vi "CRYUpdate Jump Info.vi"(8 "SourceCount":i32, 9 "MoveCount":i32, 10 "Step number Selected":i32, 11 "Action":T2(ring)) -> (0 "Jump State Out":T1(array[cluster]), 2 "Canceled?":bool)   [LabVIEW 2013]
uses:
  CRYProject Editor Global.vi
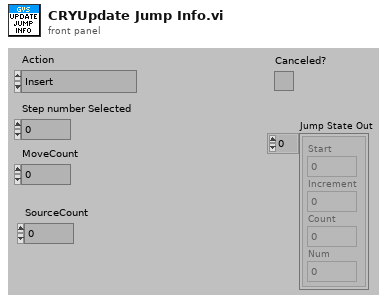
[diagram p1: front panel]
types:
  T1 = cluster{"Start":dbl, "Increment":dbl, "Count":i32, "Num":i32}[]
  T2 = enum16{"Insert", "Remove", "Move up", "Move down"}
  T3 = typedef "CRYTS.ctl" = cluster{"No.TS":u16, "TS File Path":path, "TS Name":string, "EditStepName":string, "Steps":T4[], "New State":bool, "Change State":bool, "Flattened CurveLib Data":string, "Document Data":string, "EditStepNo":u16, "Operator Start File":string, "Sequence Type":string, "Sequence Language":string}
  T4 = typedef "CRYStep.ctl" = cluster{"No.VI":i32, "Category":string, "StepName":string, "Seq setup flattened":string, "Comment":string, "Steps config.":bool[], "Jump config":i32[], "Start":dbl, "Increment":dbl, "Name":string, "Unit":string, "Y data":u16, "Y prefix":string, "Y dB ref":dbl, "Y unit":string, "Repeat State Array":cluster{"Start":dbl, "Increment":dbl, "Count":i32, "Num":i32}[]}
  T5 = enum16{"OK", "Yes", "YesNo", "YesNoCancel", "ReplaceAppend"}
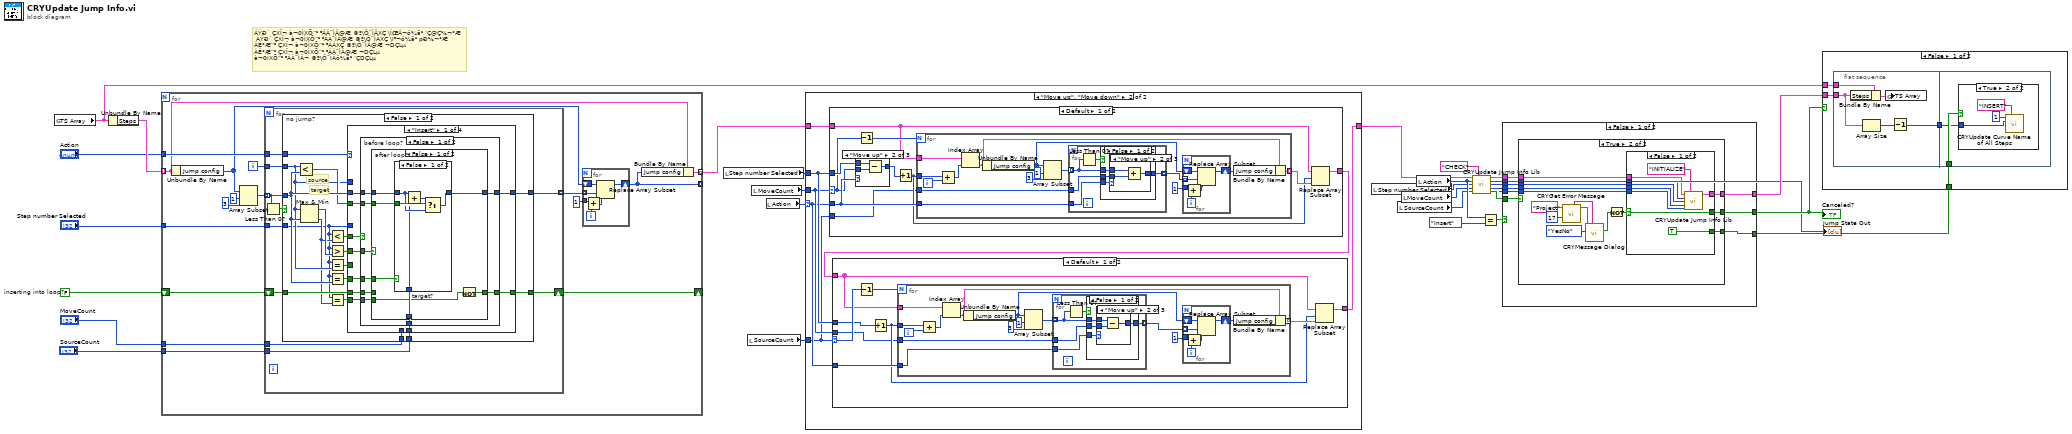
[diagram p0: block diagram]
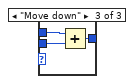
[diagram p4: hidden frame]
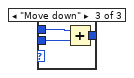
[diagram p8: hidden frame]
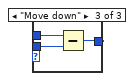
[diagram p10: hidden frame]
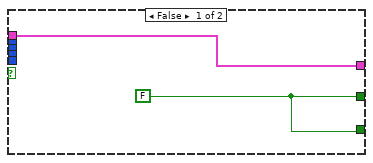
[diagram p15: hidden frame]
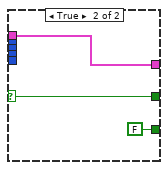
[diagram p16: hidden frame]
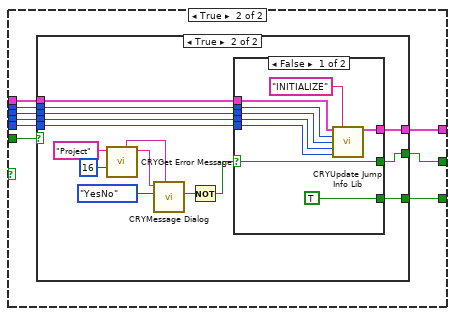
[diagram p17: hidden frame]
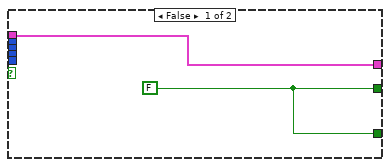
[diagram p18: hidden frame]
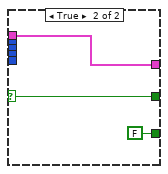
[diagram p19: hidden frame]
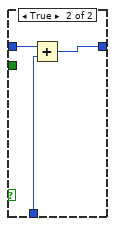
[diagram p20: hidden frame]
diagram:
  w24 = FALSE  # inserting into loop?
  # "ÁÝÐ´ ÇXÎ¬ à¬0ÌXÕ”² ³ÁÀ¨ÌÂ@Æ ©º\\Ô¨ÌÂXÇ \\ÍŒÁ¬ô¼ä² ‘Ç@Ç½¬°Æ\n ÁÝÐ´ ÇXÎ¬ à¬0ÌXÕ”² ³ÁÀ¨ÌÂ@Æ ©º\\Ô¨ÌÂXÇ \\Í³¬ô¼ä² pÐ½¬°Æ\nÀÉ°Æ”² ÇXÎ¬ à¬0ÌXÕ”² ³ÁÀXÇ ©º\\Ô¨ÌÂ@Æ ¬DÇLµ\nÀÉ°Æ”² ÇXÎ¬ à¬0ÌXÕ”² ³ÁÀ¨ÌÂ@Æ ¬DÇLµ\nà¬0ÌXÕ”² ³ÁÀ¨ÌÂ¬ ©º\\Ô¨ÌÂô¼ä² ‘ÇDÇLµ"
  n1 = global read "CRYProject Editor Global.vi" "TS Array"() -> (w23:T3)
  n2 = Unbundle By Name(w23) -> ("Steps"=w17:T4[])
  n3 = for {
    tunnel: "Step number Selected" -> [w39]
    tunnel: "Action" -> [w38]
    tunnel: [w29] -> _ mode=indexing
    tunnel: "SourceCount" -> [w35]
    shift-right: [w33] -> _
    shift-left: w24 -> [w34]
    tunnel: w17 -> [w30] mode=indexing
    tunnel: [w28] -> w21 mode=indexing
    tunnel: "MoveCount" -> [w27]
    i -> [w40]
    n4 = Unbundle By Name(w30) -> ("Jump config"=w31:i32[])
    n5 = Array Subset(array=w31, index=1, length=3) -> (w32:i32[])
    n6 = for {
      tunnel: w32 -> [w57] mode=indexing
      tunnel: w40 -> [w56]
      tunnel: w39 -> [w55]
      tunnel: w38 -> [w54]
      tunnel: [w53] -> w36 mode=indexing
      tunnel: w35 -> [w52]
      shift-right: [w51] -> w33
      shift-left: w34 -> [w50]
      tunnel: w27 -> [w49]
      n7 = Less Than 0?(x=w57) -> (x < 0?=w58:bool)
      n8 = case "no jump?" shown="False" w58 {
        tunnel: w57 -> [w70 w315]
        tunnel: w56 -> [w66 _]
        tunnel: w55 -> [w61 _]
        tunnel: w54 -> [w75 _]
        tunnel: [w73 w315] -> w53
        tunnel: w52 -> [w65 _]
        tunnel: [w64 w314] -> w51
        tunnel: w50 -> [w63 w314]
        tunnel: w49 -> [w59 _]
        frame False {
          # "target"
          # "source"
          n9 = Less?(x=w66, y=w70) -> (x < y?=w67:bool)
          n10 = Max & Min(x=w66, y=w70) -> (max(x,y)=w71:i32, min(x,y)=w62:i32)
          n11 = Less?(x=w61, y=w62) -> (x < y?=w74:bool)
          n12 = Greater?(x=w61, y=w71) -> (0:w72:bool)
          n13 = Equal?(x=w61, y=w66) -> (x = y?=w68:bool)
          n14 = Equal?(x=w61, y=w70) -> (x = y?=w69:bool)
          n15 = Equal?(x=w61, y=w62) -> (x = y?=w60:bool)
          n16 = case shown="\"Insert\"" w75 {
            tunnel: w74 -> [w85 w124 w165 w245]
            tunnel: w70 -> [w84 w123 w164 w244]
            tunnel: [w83 w122 w163 w243] -> w73
            tunnel: w72 -> [w82 w121 w162 w242]
            tunnel: w69 -> [w81 w120 w161 w241]
            tunnel: w68 -> [_ w119 w160 w240]
            tunnel: w67 -> [w80 w118 w159 w239]
            tunnel: w61 -> [_ _ w158 w238]
            tunnel: w66 -> [_ _ w157 w237]
            tunnel: w65 -> [w79 w116 w154 w234]
            tunnel: [w78 w117 w156 w236] -> w64
            tunnel: w63 -> [w77 w117 w156 w236]
            tunnel: w60 -> [w76 _ _ _]
            tunnel: w59 -> [_ _ w155 w235]
            frame "Insert" {
              n17 = case "before loop?" shown="False" w85 {
                tunnel: w84 -> [w93 w115]
                tunnel: [w92 w113] -> w83
                tunnel: w82 -> [w94 _]
                tunnel: w81 -> [w91 _]
                tunnel: w80 -> [w90 _]
                tunnel: w79 -> [w89 w114]
                tunnel: [w88 w112] -> w78
                tunnel: w77 -> [w87 w112]
                tunnel: w76 -> [w86 _]
                frame False {
                  n18 = case "after loop?" shown="False" w94 {
                    tunnel: [w100 w111] -> w92
                    tunnel: w93 -> [w99 w111]
                    tunnel: w91 -> [w101 _]
                    tunnel: w90 -> [w98 _]
                    tunnel: w89 -> [w97 _]
                    tunnel: [w95 w110] -> w88
                    tunnel: w87 -> [_ w110]
                    tunnel: w86 -> [w96 _]
                    frame False {
                      n19 = case "target?" shown="False" w101 {
                        tunnel: [w106 w108] -> w100
                        tunnel: w99 -> [w104 w109]
                        tunnel: w98 -> [w105 _]
                        tunnel: w97 -> [w102 w107]
                        frame False {
                          n20 = Add(x=w104, y=w102) -> (x+y=w103:i32)
                          n21 = Select(t=w103, s=w105, f=w104) -> (s? t:f=w106:i32)
                        }
                        frame True {
                          n22 = Add(x=w109, y=w107) -> (x+y=w108:i32)
                        }
                      }
                      n23 = Not(x=w96) -> (.not. x?=w95:bool)
                    }
                    frame True {
                    }
                  }
                }
                frame True {
                  n24 = Add(x=w115, y=w114) -> (x+y=w113:i32)
                }
              }
            }
            frame "Remove" {
              n25 = case "before loop?" shown="False" w124 {
                tunnel: w123 -> [w130 w153]
                tunnel: [w129 w151] -> w122
                tunnel: w121 -> [w131 _]
                tunnel: w120 -> [w128 _]
                tunnel: w119 -> [w127 _]
                tunnel: w118 -> [w126 _]
                tunnel: w116 -> [w125 w152]
                frame False {
                  n26 = case "after loop?" shown="False" w131 {
                    tunnel: [w136 w150] -> w129
                    tunnel: w130 -> [w135 w150]
                    tunnel: w128 -> [w137 _]
                    tunnel: w127 -> [w134 _]
                    tunnel: w126 -> [w133 _]
                    tunnel: w125 -> [w132 _]
                    frame False {
                      n27 = case "target?" shown="False" w137 {
                        tunnel: [w141 -1] -> w136
                        tunnel: w135 -> [w142 _]
                        tunnel: w134 -> [w140 _]
                        tunnel: w133 -> [w139 _]
                        tunnel: w132 -> [w138 _]
                        frame False {
                          n28 = case "source?" shown="False" w140 {
                            tunnel: [w146 -1] -> w141
                            tunnel: w142 -> [w145 _]
                            tunnel: w139 -> [w147 _]
                            tunnel: w138 -> [w144 _]
                            frame False {
                              n29 = Decrement(x=w145) -> ()  [unwired: 1 out]
                              n30 = Subtract(x=w145, y=w144) -> (x-y=w143:i32)
                              n31 = Select(t=w143, s=w147, f=w145) -> (s? t:f=w146:i32)
                            }
                            frame True {
                            }
                          }
                        }
                        frame True {
                        }
                      }
                    }
                    frame True {
                    }
                  }
                }
                frame True {
                  n32 = Decrement(x=w153) -> ()  [unwired: 1 out]
                  n33 = Subtract(x=w153, y=w152) -> (x-y=w151:i32)
                }
              }
            }
            frame "Move up" {
              n34 = case "before loop?" shown="False" w165 {
                tunnel: w164 -> [w174 w233]
                tunnel: [w173 w233] -> w163
                tunnel: w162 -> [w175 _]
                tunnel: w161 -> [w172 _]
                tunnel: w160 -> [w171 _]
                tunnel: w159 -> [w170 _]
                tunnel: w158 -> [w169 _]
                tunnel: w157 -> [w168 _]
                tunnel: w155 -> [w167 _]
                tunnel: w154 -> [w166 _]
                frame False {
                  n35 = case "after loop?" shown="False" w175 {
                    tunnel: [w183 w227] -> w173
                    tunnel: w174 -> [w182 w226]
                    tunnel: w172 -> [w184 _]
                    tunnel: w171 -> [w181 _]
                    tunnel: w170 -> [w180 _]
                    tunnel: w169 -> [w178 w230]
                    tunnel: w168 -> [w179 _]
                    tunnel: w167 -> [w177 w223]
                    tunnel: w166 -> [w176 w224]
                    frame False {
                      n36 = case "target?" shown="False" w184 {
                        tunnel: [w191 w215] -> w183
                        tunnel: w182 -> [w192 w214]
                        tunnel: w181 -> [w190 _]
                        tunnel: w180 -> [w189 _]
                        tunnel: w179 -> [w188 w219]
                        tunnel: w178 -> [w187 _]
                        tunnel: w177 -> [w186 w211]
                        tunnel: w176 -> [w185 w212]
                        frame False {
                          n37 = case "source?" shown="False" w190 {
                            tunnel: [w199 w204] -> w191
                            tunnel: w192 -> [w197 w205]
                            tunnel: w189 -> [_ _]
                            tunnel: w188 -> [_ w206]
                            tunnel: w187 -> [w198 _]
                            tunnel: w186 -> [w194 _]
                            tunnel: w185 -> [w195 _]
                            frame False {
                              n38 = Decrement(x=w198) -> (x-1=w201:i32)
                              n39 = Increment(x=w197) -> ()  [unwired: 1 out]
                              n40 = Equal?(x=w201, y=w197) -> (x = y?=w200:bool)
                              n41 = case shown="Default" w195 {
                                selector: w195 -> [w202 _]
                                tunnel: [w202 w203] -> w193
                                tunnel: w194 -> [_ w203]
                                frame Default {
                                }
                                frame 1 {
                                }
                              }
                              n42 = Add(x=w197, y=w193) -> (x+y=w196:i32)
                              n43 = Select(t=w196, s=w200, f=w197) -> (s? t:f=w199:i32)
                            }
                            frame True {
                              n44 = Decrement(x=w206) -> (x-1=w209:i32)
                              n45 = Equal?(x=w209, y=w205) -> (x = y?=w207:bool)
                              n46 = Select(t=-1, s=w207, f=w205) -> (s? t:f=w204:i32)
                            }
                          }
                        }
                        frame True {
                          n47 = Increment(x=w219) -> (x+1=w218:i32)
                          n48 = Equal?(x=w218, y=w214) -> (x = y?=w216:bool)
                          n49 = Decrement(x=w214) -> ()  [unwired: 1 out]
                          n50 = case shown="1" w212 {
                            selector: w212 -> [w220 _]
                            tunnel: [w220 w221] -> w210
                            tunnel: w211 -> [_ w221]
                            frame Default {
                            }
                            frame 1 {
                            }
                          }
                          n51 = Subtract(x=w214, y=w210) -> (x-y=w213:i32)
                          n52 = Select(t=-1, s=w216, f=w213) -> (s? t:f=w215:i32)
                        }
                      }
                    }
                    frame True {
                      n53 = Decrement(x=w230) -> (x-1=w229:i32)
                      n54 = Equal?(x=w226, y=w229) -> (x = y?=w228:bool)
                      n55 = Increment(x=w226) -> ()  [unwired: 1 out]
                      n56 = case shown="1" w224 {
                        selector: w224 -> [w231 _]
                        tunnel: [w231 w232] -> w222
                        tunnel: w223 -> [_ w232]
                        frame Default {
                        }
                        frame 1 {
                        }
                      }
                      n57 = Add(x=w226, y=w222) -> (x+y=w225:i32)
                      n58 = Select(t=w225, s=w228, f=w226) -> (s? t:f=w227:i32)
                    }
                  }
                }
                frame True {
                }
              }
            }
            frame "Move down" {
              n59 = case "before loop?" shown="False" w245 {
                tunnel: w244 -> [w254 w307]
                tunnel: [w253 w308] -> w243
                tunnel: w242 -> [w255 _]
                tunnel: w241 -> [w252 _]
                tunnel: w240 -> [w251 _]
                tunnel: w239 -> [w250 _]
                tunnel: w238 -> [w249 w309]
                tunnel: w237 -> [w248 _]
                tunnel: w235 -> [w247 w304]
                tunnel: w234 -> [w246 w305]
                frame False {
                  n60 = case "after loop?" shown="False" w255 {
                    tunnel: [w263 w302] -> w253
                    tunnel: w254 -> [w262 w302]
                    tunnel: w252 -> [w264 _]
                    tunnel: w251 -> [w261 _]
                    tunnel: w250 -> [w260 _]
                    tunnel: w249 -> [w258 _]
                    tunnel: w248 -> [w259 _]
                    tunnel: w247 -> [w257 _]
                    tunnel: w246 -> [w256 _]
                    frame False {
                      n61 = case "target?" shown="False" w264 {
                        tunnel: [w271 w295] -> w263
                        tunnel: w262 -> [w272 w294]
                        tunnel: w261 -> [w270 _]
                        tunnel: w260 -> [w269 _]
                        tunnel: w259 -> [w268 w299]
                        tunnel: w258 -> [w267 _]
                        tunnel: w257 -> [w266 w291]
                        tunnel: w256 -> [w265 w292]
                        frame False {
                          n62 = case "source?" shown="False" w270 {
                            tunnel: [w279 w284] -> w271
                            tunnel: w272 -> [w277 w285]
                            tunnel: w269 -> [_ _]
                            tunnel: w268 -> [_ w286]
                            tunnel: w267 -> [w278 _]
                            tunnel: w266 -> [w274 _]
                            tunnel: w265 -> [w275 _]
                            frame False {
                              n63 = Increment(x=w278) -> (x+1=w281:i32)
                              n64 = Decrement(x=w277) -> ()  [unwired: 1 out]
                              n65 = Equal?(x=w281, y=w277) -> (x = y?=w280:bool)
                              n66 = case shown="1" w275 {
                                selector: w275 -> [w282 _]
                                tunnel: [w282 w283] -> w273
                                tunnel: w274 -> [_ w283]
                                frame Default {
                                }
                                frame 1 {
                                }
                              }
                              n67 = Subtract(x=w277, y=w273) -> (x-y=w276:i32)
                              n68 = Select(t=w276, s=w280, f=w277) -> (s? t:f=w279:i32)
                            }
                            frame True {
                              n69 = Increment(x=w286) -> (x+1=w289:i32)
                              n70 = Equal?(x=w289, y=w285) -> (x = y?=w287:bool)
                              n71 = Select(t=-1, s=w287, f=w285) -> (s? t:f=w284:i32)
                            }
                          }
                        }
                        frame True {
                          n72 = Decrement(x=w299) -> (x-1=w298:i32)
                          n73 = Equal?(x=w298, y=w294) -> (x = y?=w296:bool)
                          n74 = case shown="1" w292 {
                            selector: w292 -> [w300 _]
                            tunnel: [w300 w301] -> w290
                            tunnel: w291 -> [_ w301]
                            frame Default {
                            }
                            frame 1 {
                            }
                          }
                          n75 = Increment(x=w294) -> ()  [unwired: 1 out]
                          n76 = Add(x=w294, y=w290) -> (x+y=w293:i32)
                          n77 = Select(t=-1, s=w296, f=w293) -> (s? t:f=w295:i32)
                        }
                      }
                    }
                    frame True {
                    }
                  }
                }
                frame True {
                  n78 = Increment(x=w309) -> (x+1=w311:i32)
                  n79 = Equal?(x=w307, y=w311) -> (x = y?=w310:bool)
                  n80 = Decrement(x=w307) -> ()  [unwired: 1 out]
                  n81 = case shown="1" w305 {
                    selector: w305 -> [w312 _]
                    tunnel: [w312 w313] -> w303
                    tunnel: w304 -> [_ w313]
                    frame Default {
                    }
                    frame 1 {
                    }
                  }
                  n82 = Subtract(x=w307, y=w303) -> (x-y=w306:i32)
                  n83 = Select(t=w306, s=w310, f=w307) -> (s? t:f=w308:i32)
                }
              }
            }
          }
        }
        frame True {
        }
      }
    }
    n84 = for {
      tunnel: 1 -> [w46]
      tunnel: w36 -> [w45] mode=indexing
      shift-right: [w43] -> w29
      shift-left: w31 -> [w44]
      i -> [w48]
      n85 = Add(x=w46, y=w48) -> (x+y=w47:i32)
      n86 = Replace Array Subset(array=w44, new element=w45, index=w47) -> (w43:i32[])
    }
    n87 = Bundle By Name(cluster=w30, "Jump config"=w29) -> (w28:T4)
  }
  n88 = local read "Step number Selected"() -> (w20:i32)
  n89 = local read "SourceCount"() -> (w18:i32)
  n90 = local read "MoveCount"() -> (w19:i32)
  n91 = local read "Action"() -> (w22:T2)
  n92 = case shown="\"Move up\", \"Move down\"" w22 {
    selector: w22 -> [_ w318]
    tunnel: w21 -> [w316 w323]
    tunnel: w20 -> [_ w321]
    tunnel: w19 -> [_ w319]
    tunnel: w18 -> [_ w317]
    tunnel: [w316 w320] -> w4
    frame Default {
    }
    frame "Move up", "Move down" {
      n93 = case shown="Default" w319 {
        selector: w319 -> [w377 _]
        tunnel: w323 -> [w374 w424]
        tunnel: w321 -> [w378 _]
        tunnel: [w375 w424] -> w322
        tunnel: w318 -> [w379 _]
        tunnel: w317 -> [w371 _]
        frame Default {
          n94 = case shown="\"Move up\"" w379 {
            tunnel: w378 -> [_ w383 w386]
            tunnel: w377 -> [_ w382 w385]
            tunnel: [_ w381 w384] -> w376
            frame Default {
            }
            frame "Move up" {
              n95 = Subtract(x=w383, y=w382) -> (x-y=w381:i32)
            }
            frame "Move down" {
              n96 = Add(x=w386, y=w385) -> (x+y=w384:i32)
            }
          }
          n97 = Decrement(x=w377) -> (x-1=w380:i32)
          n98 = Increment(x=w376) -> (x+1=w372:i32)
          n99 = for {
            N: w380 -> [_]
            tunnel: w374 -> [w401]
            tunnel: w371 -> [w397]
            tunnel: [w391] -> w373 mode=indexing
            tunnel: w372 -> [w390]
            tunnel: w379 -> [w387]
            i -> [w389]
            n100 = Add(x=w390, y=w389) -> (x+y=w388:i32)
            n101 = Index Array(array=w401, index=w388) -> (element=w392:T4)
            n102 = Unbundle By Name(w392) -> ("Jump config"=w396:i32[])
            n103 = Array Subset(array=w396, index=1, length=3) -> (w398:i32[])
            n104 = for {
              tunnel: w398 -> [w409] mode=indexing
              tunnel: w397 -> [w412]
              tunnel: [w411] -> w395 mode=indexing
              tunnel: w387 -> [w410]
              n105 = Less Than 0?(x=w409) -> (x < 0?=w408:bool)
              n106 = case shown="False" w408 {
                tunnel: w409 -> [w416 w423]
                tunnel: w412 -> [w415 _]
                tunnel: [w414 w423] -> w411
                tunnel: w410 -> [w413 _]
                frame False {
                  n107 = case shown="\"Move up\"" w413 {
                    tunnel: w416 -> [_ w419 w422]
                    tunnel: w415 -> [_ w418 w421]
                    tunnel: [_ w417 w420] -> w414
                    frame Default {
                    }
                    frame "Move up" {
                      n108 = Add(x=w419, y=w418) -> (x+y=w417:i32)
                    }
                    frame "Move down" {
                      n109 = Subtract(x=w422, y=w421) -> (x-y=w420:i32)
                    }
                  }
                }
                frame True {
                }
              }
            }
            n110 = for {
              tunnel: 1 -> [w405]
              tunnel: w395 -> [w404] mode=indexing
              shift-right: [w402] -> w393
              shift-left: w396 -> [w403]
              i -> [w407]
              n111 = Add(x=w405, y=w407) -> (x+y=w406:i32)
              n112 = Replace Array Subset(array=w403, new element=w404, index=w406) -> (w402:i32[])
            }
            n113 = Bundle By Name(cluster=w392, "Jump config"=w393) -> (w391:T4)
          }
          n114 = Replace Array Subset(array=w374, new element=w373, index=w372) -> (w375:T4[])
        }
        frame 1 {
        }
      }
      n115 = case shown="Default" w317 {
        selector: w317 -> [w331 _]
        tunnel: w322 -> [w328 w370]
        tunnel: w321 -> [w330 _]
        tunnel: [w326 w370] -> w320
        tunnel: w318 -> [w329 _]
        tunnel: w319 -> [w324 _]
        frame Default {
          n116 = Decrement(x=w331) -> (x-1=w332:i32)
          n117 = Increment(x=w330) -> (x+1=w325:i32)
          n118 = for {
            N: w332 -> [_]
            tunnel: w328 -> [w347]
            tunnel: w324 -> [w343]
            tunnel: [w337] -> w327 mode=indexing
            tunnel: w325 -> [w336]
            tunnel: w329 -> [w333]
            i -> [w335]
            n119 = Add(x=w336, y=w335) -> (x+y=w334:i32)
            n120 = Index Array(array=w347, index=w334) -> (element=w338:T4)
            n121 = Unbundle By Name(w338) -> ("Jump config"=w342:i32[])
            n122 = Array Subset(array=w342, index=1, length=3) -> (w344:i32[])
            n123 = for {
              tunnel: w344 -> [w355] mode=indexing
              tunnel: w343 -> [w358]
              tunnel: [w357] -> w341 mode=indexing
              tunnel: w333 -> [w356]
              n124 = Less Than 0?(x=w355) -> (x < 0?=w354:bool)
              n125 = case shown="False" w354 {
                tunnel: w358 -> [w362 _]
                tunnel: [w361 w369] -> w357
                tunnel: w356 -> [w360 _]
                tunnel: w355 -> [w359 w369]
                frame False {
                  n126 = case shown="\"Move up\"" w360 {
                    tunnel: w359 -> [_ w365 w368]
                    tunnel: w362 -> [_ w364 w367]
                    tunnel: [_ w363 w366] -> w361
                    frame Default {
                    }
                    frame "Move up" {
                      n127 = Subtract(x=w365, y=w364) -> (x-y=w363:i32)
                    }
                    frame "Move down" {
                      n128 = Add(x=w368, y=w367) -> (x+y=w366:i32)
                    }
                  }
                }
                frame True {
                }
              }
            }
            n129 = for {
              tunnel: 1 -> [w351]
              tunnel: w341 -> [w350] mode=indexing
              shift-right: [w348] -> w339
              shift-left: w342 -> [w349]
              i -> [w353]
              n130 = Add(x=w351, y=w353) -> (x+y=w352:i32)
              n131 = Replace Array Subset(array=w349, new element=w350, index=w352) -> (w348:i32[])
            }
            n132 = Bundle By Name(cluster=w338, "Jump config"=w339) -> (w337:T4)
          }
          n133 = Replace Array Subset(array=w328, new element=w327, index=w325) -> (w326:T4[])
        }
        frame 1 {
        }
      }
    }
  }
  n134 = local read "Step number Selected"() -> (w7:i32)
  n135 = local read "SourceCount"() -> (w5:i32)
  n136 = local read "MoveCount"() -> (w6:i32)
  n137 = local read "Action"() -> (w9:T2)
  n138 = call "CRYUpdate Jump Info Lib.vi"("Steps In"=w4, "sOption"="CHECK", "Action"=w9, "Step number Selected"=w7, "MoveCount"=w6, "SourceCount"=w5) -> ("Steps Out"=w8:T4[], "Jump State Out"=→"Jump State Out":T1, "Canceled?"=w11:bool)  [unwired: 7 in]
  n139 = Equal?(x=w9, y=T2."Insert") -> (x = y?=w26:bool)
  n140 = case shown="False" w26 {
    tunnel: [w433 w471] -> w10
    tunnel: w11 -> [w432 w470]
    tunnel: w9 -> [w431 w468]
    tunnel: w8 -> [w430 w469]
    tunnel: w7 -> [w429 w467]
    tunnel: w6 -> [w428 w466]
    tunnel: w5 -> [w427 w465]
    tunnel: [w426 w464] -> w3
    tunnel: [w425 w463] -> w1
    frame False {
      n141 = case shown="True" w432 {
        tunnel: [w434 w443] -> w433
        tunnel: w431 -> [_ w442]
        tunnel: w430 -> [w435 w441]
        tunnel: w429 -> [_ w440]
        tunnel: w428 -> [_ w439]
        tunnel: w427 -> [_ w438]
        tunnel: [w435 w437] -> w426
        tunnel: [w434 w436] -> w425
        frame False {
          w434 = FALSE
        }
        frame True {
          n142 = call "CRYGet Error Message.vi"("Error No"=17, "Kind"="Project") -> ("Message"=w450:string, "Window Title"=w448:string)  [unwired: 4 in, 4 out]
          n143 = call "CRYMessage Dialog.vi"("Window Title"=w448, "YesNoCancel"=T5."YesNo", "Message Content"=w450) -> ("YesNo"=w445:bool)  [unwired: 7 in, 1 out]
          n144 = Not(x=w445) -> (.not. x?=w444:bool)
          n145 = case shown="False" w444 {
            selector: w444 -> [w459 w462]
            tunnel: [w459 w462] -> w443
            tunnel: w442 -> [w457 _]
            tunnel: w441 -> [w456 w461]
            tunnel: w440 -> [w455 _]
            tunnel: w439 -> [w454 _]
            tunnel: w438 -> [w453 _]
            tunnel: [w452 w461] -> w437
            tunnel: [TRUE FALSE] -> w436
            frame False {
              n146 = call "CRYUpdate Jump Info Lib.vi"("Steps In"=w456, "sOption"="INITIALIZE", "Action"=w457, "Step number Selected"=w455, "MoveCount"=w454, "SourceCount"=w453) -> ("Steps Out"=w452:T4[])  [unwired: 7 in, 2 out]
            }
            frame True {
            }
          }
        }
      }
    }
    frame True {
      n147 = case shown="True" w470 {
        tunnel: [w472 w481] -> w471
        tunnel: w469 -> [w473 w480]
        tunnel: w468 -> [_ w479]
        tunnel: w467 -> [_ w478]
        tunnel: w466 -> [_ w477]
        tunnel: w465 -> [_ w476]
        tunnel: [w473 w475] -> w464
        tunnel: [w472 w474] -> w463
        frame False {
          w472 = FALSE
        }
        frame True {
          n148 = call "CRYGet Error Message.vi"("Error No"=16, "Kind"="Project") -> ("Message"=w488:string, "Window Title"=w486:string)  [unwired: 4 in, 4 out]
          n149 = call "CRYMessage Dialog.vi"("Window Title"=w486, "YesNoCancel"=T5."YesNo", "Message Content"=w488) -> ("YesNo"=w483:bool)  [unwired: 7 in, 1 out]
          n150 = Not(x=w483) -> (.not. x?=w482:bool)
          n151 = case shown="False" w482 {
            selector: w482 -> [w497 w500]
            tunnel: [w497 w500] -> w481
            tunnel: w479 -> [w495 _]
            tunnel: w480 -> [w494 w499]
            tunnel: w478 -> [w493 _]
            tunnel: w477 -> [w492 _]
            tunnel: w476 -> [w491 _]
            tunnel: [w490 w499] -> w475
            tunnel: [TRUE FALSE] -> w474
            frame False {
              n152 = call "CRYUpdate Jump Info Lib.vi"("Steps In"=w494, "sOption"="INITIALIZE", "Action"=w495, "Step number Selected"=w493, "MoveCount"=w492, "SourceCount"=w491) -> ("Steps Out"=w490:T4[])  [unwired: 7 in, 2 out]
            }
            frame True {
            }
          }
        }
      }
    }
  }
  "Canceled?" <- w10
  n153 = case shown="False" w10 {
    tunnel: w23 -> [w504 _]
    tunnel: w3 -> [w503 _]
    tunnel: w1 -> [w502 _]
    frame False {
      n154 = flat-sequence {
        tunnel: w504 -> [w509]
        tunnel: w503 -> [w507]
        tunnel: [w505] -> w501
        tunnel: w502 -> [w511]
        tunnel: w501 -> [w510]
        frame #0 {
          n155 = Bundle By Name(cluster=w509, "Steps"=w507) -> (w508:T3)
          n156 = Array Size(array=w507) -> (size(s)=w506:i32)
          n157 = global write "CRYProject Editor Global.vi" "TS Array"(w508) -> ()
          n158 = Decrement(x=w506) -> (x-1=w505:i32)
        }
        frame #1 {
          n159 = case shown="True" w511 {
            tunnel: w510 -> [_ w512]
            frame False {
            }
            frame True {
              n160 = call "CRYUpdate Curve Name of All Steps.vi"("Start Index"=1, "sOption"="INSERT", "End Index"=w512) -> ()  [unwired: 13 in]
            }
          }
        }
      }
    }
    frame True {
    }
  }
